vi "DN4_GetSamples.vi"(1 "Task ID":u32) -> (0 "samples":i32)   [LabVIEW 2009]
uses:
  Windows/System32/AdvLvDaq.dll
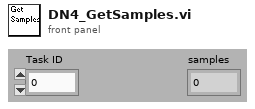
[diagram p1: front panel]
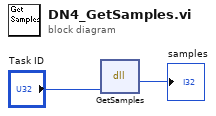
[diagram p0: block diagram]
diagram:
  n1 = dll-call lib="C:/Windows/System32/AdvLvDaq.dll" fn="GetSamples"("taskId"="Task ID") -> ("return type"=→"samples":i32)  [unwired: 4 in, 2 out]
